vi "qJAX.vi"(0 "System no.":i32=1 min=1 max=4 step=1, 1 "JoystickID to query":i32[](array[numeric]), 2 "Joystick axis":i32[](array[numeric]), 3 "Without JoystickIDs?":bool, 5 "error in":errorcluster) -> (14 "Controlled axes":string[](array[string]), 19 "error out":errorcluster)   [LabVIEW 2026]
doc: "Returns which axes are assigned to be controlled by joystick axes of joysticks connected to the controller.\n\nE-709: Only supported if E-709 is used inside C-867K012/K013."
panel:
  # "Returns which axes are assigned to be controlled  by joystick axes of joysticks connected to \nthe controller."
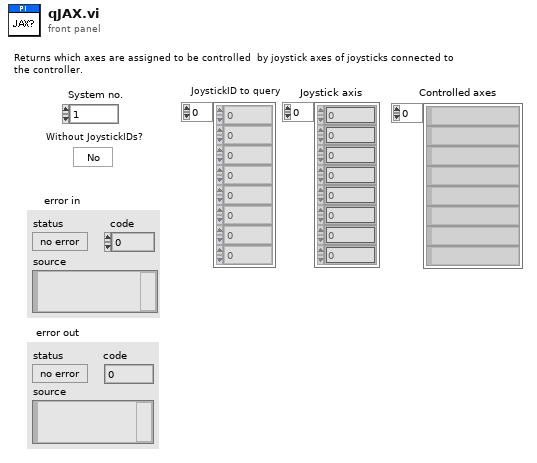
[diagram p1: front panel]
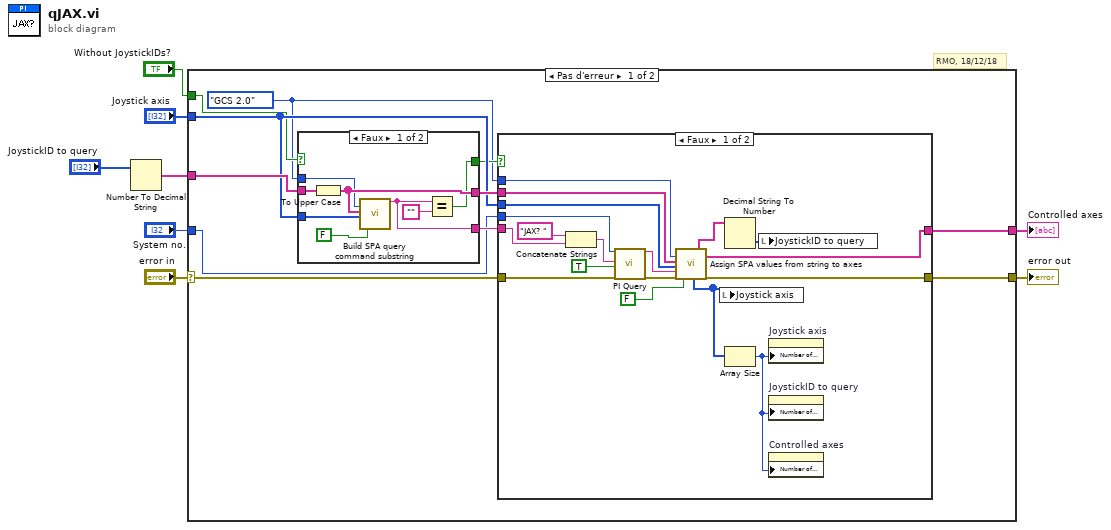
[diagram p0: block diagram]
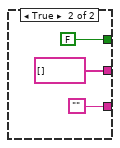
[diagram p2: hidden frame]
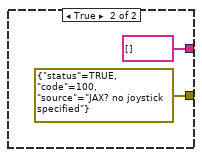
[diagram p3: hidden frame]
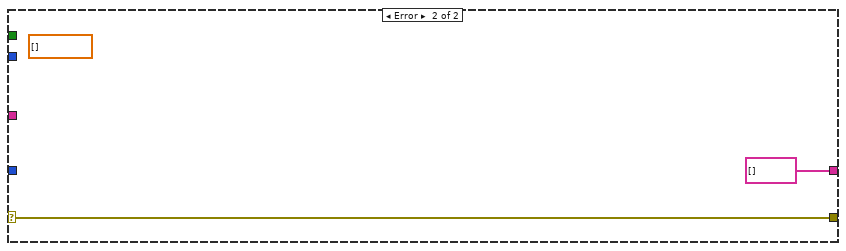
[diagram p4: hidden frame]
diagram:
  # "RMO, 18/12/18"
  n1 = Number To Decimal String(number="JoystickID to query") -> (decimal integer string=w4:string[])  [unwired: 1 out]
  n2 = case shown="Pas d'erreur" "error in" {
    selector: "error in" -> [w9 w51]
    tunnel: w4 -> [w19 _]
    tunnel: "System no." -> [w11 _]
    tunnel: "Joystick axis" -> [w16 _]
    tunnel: [w15 w51] -> w6
    tunnel: "Without JoystickIDs?" -> [w13 _]
    tunnel: [w12 string[] [] ("Parameter strings")] -> w2
    frame No Error {
      w10 = enum16{"GCS 1.0", "GCS 2.0"}."GCS 2.0" ("Syntax")
      n3 = case shown="Faux" w13 {
        tunnel: w19 -> [w27 _]
        tunnel: [w26 "" ("Command substring")] -> w18
        tunnel: [w25 string[] [] ("Designator to query")] -> w17
        tunnel: w16 -> [w24 _]
        tunnel: [w23 FALSE] -> w14
        tunnel: w10 -> [w22 _]
        frame False {
          n4 = To Upper Case(1:w27) -> (0:w25:string[])
          n5 = call "Build SPA query command substring.vi"("Syntax"=w22, "Axes to query"=w25, "Parameter number"=w24, "Parameter no. format \n(Decimal: FALSE)"=FALSE ("Parameter no. format \n(Decimal: FALSE)")) -> ("Command substring"=w26:string)  [unwired: 3 in, 12 out]
          n6 = Equal?(x=w26, y="" ("x")) -> (x = y?=w23:bool)
        }
        frame True {
        }
      }
      n7 = case shown="Faux" w14 {
        tunnel: w9 -> [w41 _]
        tunnel: w18 -> [w45 _]
        tunnel: w17 -> [w44 _]
        tunnel: w11 -> [w40 _]
        tunnel: w16 -> [w43 _]
        tunnel: [w37 errorcluster {"status"=TRUE, "code"=100, "source"="JAX? no joystick specified"} ("error out")] -> w15
        tunnel: [w42 string[] [] ("Parameter strings")] -> w12
        tunnel: w10 -> [w39 _]
        frame False {
          n8 = Concatenate Strings("JAX? ", w45) -> (w46:string)
          n9 = call "PI Query.vi"("System no."=w40, "String to send"=w46, "Attach termination char.?"=TRUE ("Attach Linefeed?"), "error in"=w41) -> ("String read"=w31:string, "error out"=w32:errorcluster)  [unwired: 3 in, 11 out]
          n10 = call "Assign SPA values from string to axes.vi"("Syntax"=w39, "Queried axes"=w44, "Parameter no."=w43, "Input string"=w31, "error in"=w32, "Parameter no. format \n(Decimal: FALSE)"=FALSE ("Parameter no. format \n(Decimal: FALSE)")) -> ("Parameter no. out"=w34:i32[], "Queried axes out"=w36:string[], "Parameter strings"=w42:string[], "error out"=w37:errorcluster)  [unwired: 2 in, 8 out]
          n11 = local write "Joystick axis"(w34) -> ()
          n12 = Decimal String To Number(string=w36) -> (number=w35:i32[])  [unwired: 3 out]
          n13 = Array Size(array=w34) -> (size(s)=w33:i32)
          n14 = local write "JoystickID to query"(w35) -> ()
          n15 = property on="Joystick axis" class="Tabl (strict)"("Number of Rows"=w33) -> ()  [unwired: 2 in, 2 out]
          n16 = property on="JoystickID to query" class="Tabl (strict)"("Number of Rows"=w33) -> ()  [unwired: 2 in, 2 out]
          n17 = property on="Controlled axes" class="Tabl (strict)"("Number of Rows"=w33) -> ()  [unwired: 2 in, 2 out]
        }
        frame True {
        }
      }
    }
    frame Error {
      (unwired) dbl[] [] ("Parameter values")
    }
  }
  "error out" <- w6
  "Controlled axes" <- w2
